vi "SPARC Settings 3.1.vi"(8 "error in (no error)":errorcluster) -> (0 "error out":errorcluster)   [LabVIEW 2020]
panel:
  in  "OK Button":bool
  in  "Pad Level":dbl
  in  "Amplitude Threshold":dbl=0.01 min=0.01 max=0.05 step=0.01 format="%#.2g"
  in  "Cut-off Frequency (Hz)":dbl=1.0 min=1.0 max=50.0 step=0.5 format="%#.1g"
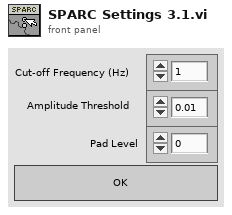
[diagram p1: front panel]
types:
  T1 = enum16{"open", "replace", "create", "open or create", "replace or create", "replace or create with confirmation"}
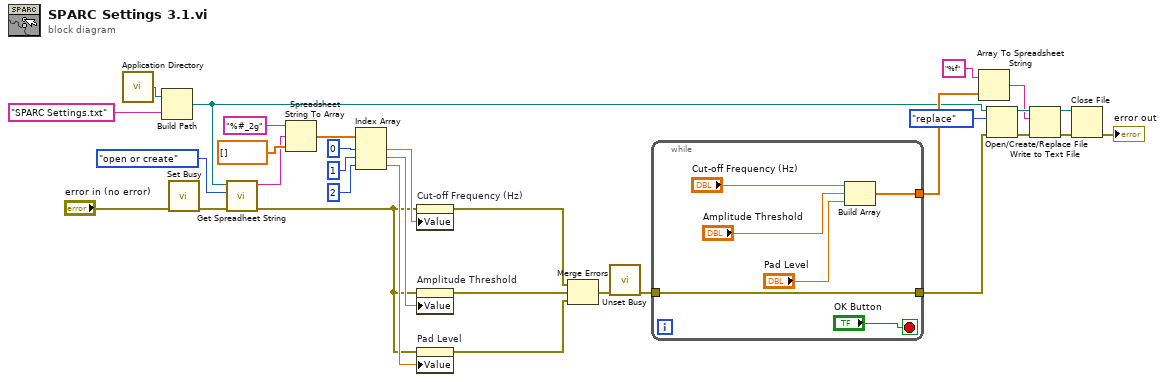
[diagram p0: block diagram]
diagram:
  n1 = call <vilib>:"Application Directory.vi"() -> ("Application Directory"=w29:path)
  n2 = Build Path(base path=w29, name or relative path="SPARC Settings.txt") -> (appended path=w5:path)
  n3 = call <vilib>:"Set Busy.vi"("error in (no error)"="error in (no error)") -> ("error out"=w2:errorcluster)  [unwired: 9 in, 1 out]
  n4 = call "Get Spreadheet String.vi"("error in (no error)"=w2, "operation (0:open)"=T1."open or create", "File Path"=w5) -> ("error out"=w3:errorcluster, "Spreadsheet String"=w4:string)  [unwired: 7 in]
  n5 = Spreadsheet String To Array(format string="%#_2g", spreadsheet string=w4, array type (2D Dbl)=dbl[] []) -> (array=w26:dbl[])  [unwired: 1 in]
  n6 = Index Array(array=w26, index #1=0 ("index"), index #2=1 ("index"), index #3=2 ("index")) -> (element #1=w22:dbl, element #2=w21:dbl, element #3=w20:dbl)
  n7 = property on="Cut-off Frequency (Hz)" class="DigNum (strict)"(error in=w3, "Value"=w22) -> (error out=w18:errorcluster)  [unwired: 1 in, 1 out]
  n8 = property on="Amplitude Threshold" class="DigNum (strict)"(error in=w3, "Value"=w21) -> (error out=w17:errorcluster)  [unwired: 1 in, 1 out]
  n9 = property on="Pad Level" class="DigNum (strict)"(error in=w3, "Value"=w20) -> (error out=w16:errorcluster)  [unwired: 1 in, 1 out]
  n10 = Merge Errors(w18, w17, w16) -> (w11:errorcluster)
  n11 = call <vilib>:"Unset Busy.vi"("error in (no error)"=w11) -> ("error out"=w10:errorcluster)  [unwired: 10 in]
  n12 = while {
    tunnel: [w37] -> w15
    tunnel: w10 -> [w37]
    tunnel: [w33] -> w6
    stop <- "OK Button" stop-if-true
    n13 = Build Array("Cut-off Frequency (Hz)", "Amplitude Threshold", "Pad Level") -> (w33:dbl[])
  }
  n14 = Array To Spreadsheet String(array=w6, 3:"%f" ("format string")) -> (spreadsheet string=w7:string)  [unwired: 1 in]
  n15 = Open/Create/Replace File(file path (use dialog)=w5, error in=w15, operation (0:open)=T1."replace") -> (refnum out=w13:refnum<file>, error out=w14:errorcluster)  [unwired: 3 in, 1 out]
  n16 = Write to Text File(file (use dialog)=w13, text=w7, error in=w14) -> (refnum out=w31:refnum<file>, error out=w32:errorcluster)  [unwired: 1 in, 1 out]
  n17 = Close File(refnum=w31, error in=w32) -> (error out=→"error out":errorcluster)  [unwired: 1 out]
